vi "Output Distance.vi"(8 "error in (no error)":errorcluster) -> (0 "error out":errorcluster, 3 "distance":dbl(slide)=125.0 scale=0.0..250.0 scale format="%3d")   [LabVIEW 2013]
panel:
  in  "Scaling factor (s/in)":dbl=0.000147
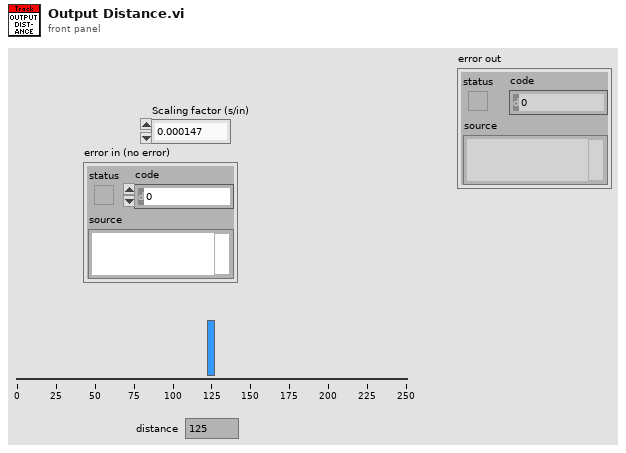
[diagram p1: front panel]
types:
  T1 = typedef "WPI_CounterDevRef.ctl" = cluster{"DevStatus":errorcluster, "CntIndex":T2}
  T2 = typedef "FPGA_CounterCtrSystemIndex.ctl" = enum8{"Ctr 0", "Ctr 1", "Ctr 2", "Ctr 3", "Ctr 4", "Ctr 5", "Ctr 6", "Ctr 7", "Invalid"}
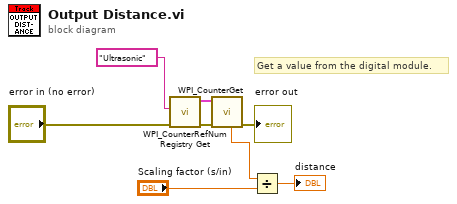
[diagram p0: block diagram]
diagram:
  # "Get a value from the digital module."
  n1 = call <vilib>:"WPI_CounterRefNum Registry Get.vi"("error in (no error)"="error in (no error)", "refnum name"="Ultrasonic") -> ("error out"=w3:errorcluster, "CounterDevRef"=w4:T1)  [unwired: 8 in]
  n2 = call <vilib>:"WPI_CounterGet.vi"("error in (no error)"=w3, "CounterDevRef in"=w4) -> ("error out"=→"error out":errorcluster, "Period (sec)"=w7:dbl)  [unwired: 4 in, 4 out]
  n3 = Divide(x=w7, y="Scaling factor (s/in)") -> (x/y=→"distance":dbl)
